vi "pmu_Check Name Length.vi"(8 "error in (no error)":errorcluster, 11 "name in":string) -> (0 "error out":errorcluster, 3 "name out":string)   [LabVIEW 2011, in "NI_EP_PMU.lvlib"]
uses:
  <vilib>/addons/Electrical Power/PMU/NI_EP_PMU.lvlib
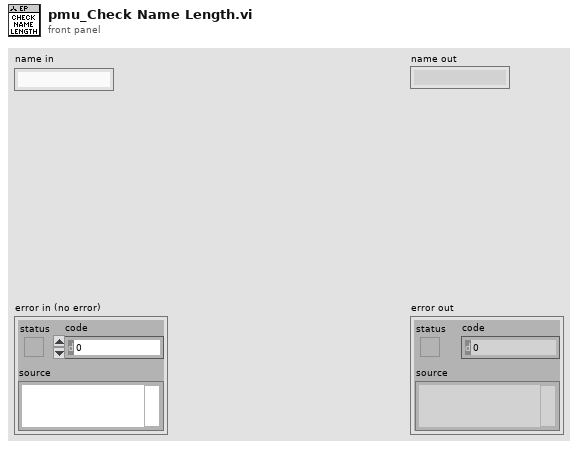
[diagram p1: front panel]
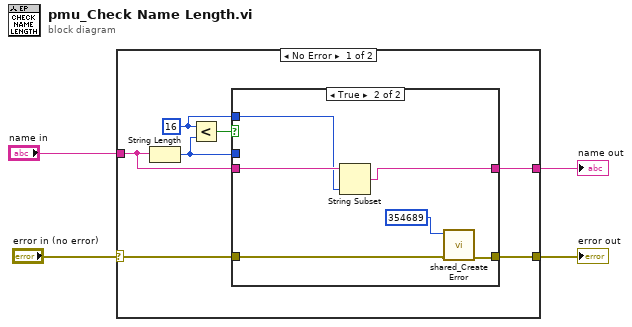
[diagram p0: block diagram]
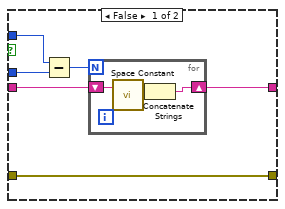
[diagram p2: hidden frame]
diagram:
  n1 = case shown="No Error" "error in (no error)" {
    selector: "error in (no error)" -> [w10 w27]
    tunnel: [w9 w27] -> w3
    tunnel: "name in" -> [w6 _]
    tunnel: [w5 _] -> w1
    frame No Error {
      w7 = 16 ("y")
      n2 = String Length(string=w6) -> (length=w8:i32)
      n3 = Less?(x=w7, y=w8) -> (x < y?=w11:bool)
      n4 = case shown="True" w11 {
        tunnel: w10 -> [w17 w22]
        tunnel: [w17 w21] -> w9
        tunnel: w8 -> [w13 _]
        tunnel: w7 -> [w15 w25]
        tunnel: w6 -> [w14 w26]
        tunnel: [w12 w24] -> w5
        frame False {
          n5 = Subtract(x=w15, y=w13) -> (x-y=w16:i32)
          n6 = for {
            N: w16 -> [_]
            shift-right: [w18] -> w12
            shift-left: w14 -> [w19]
            n7 = call <vilib>:"Space Constant.vi"() -> ("String"=w20:string)
            n8 = Concatenate Strings(w19, w20) -> (w18:string)
          }
        }
        frame True {
          n9 = String Subset(string=w26, length (rest)=w25) -> (substring=w24:string)  [unwired: 1 in]
          n10 = call <vilib>:"shared_Create Error.vi"("error in (no error)"=w22, "error code (0)"=354689) -> ("error out"=w21:errorcluster)  [unwired: 9 in]
        }
      }
    }
    frame Error {
    }
  }
  "error out" <- w3
  "name out" <- w1
